vi "DAQNavi Create Channel(CO-Pulse Width).vi"(0 "task in":i32=-1, 5 "physical channels":string="DemoDevice,BID#0/cntr0", 7 "high period":dbl=-1.0, 9 "low period":dbl=-1.0, 11 "error in (no error)":errorcluster) -> (4 "task out":i32, 15 "error out":errorcluster)   [LabVIEW 2020]
uses:
  DAQNavi_LV.dll
panel:
  in  "pulse width 2":cluster{"high period":dbl, "low period":dbl}
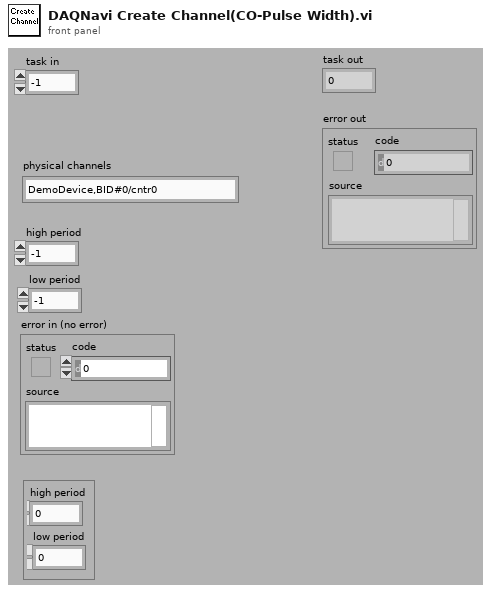
[diagram p1: front panel]
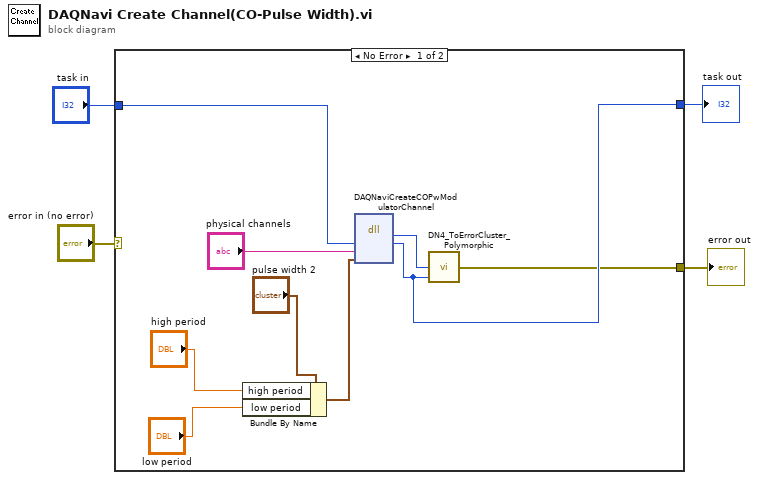
[diagram p0: block diagram]
diagram:
  n1 = case shown="No Error" "error in (no error)" {
    selector: "error in (no error)" -> [_ w14]
    tunnel: "task in" -> [w13 w15]
    tunnel: [w6 w15] -> w2
    tunnel: [w5 w14] -> w1
    frame No Error {
      n2 = Bundle By Name(cluster="pulse width 2", "high period"="high period", "low period"="low period") -> (w7:cluster{"high period":dbl, "low period":dbl})
      n3 = dll-call lib="DAQNavi_LV.dll" fn="DAQNaviCreateCOPwModulatorChannel"("taskID"=w13, "physicalChannel"="physical channels", "pulseWidth"=w7) -> ("return type"=w11:i32, "taskID"=w6:i32)  [unwired: 5 in, 2 out]
      n4 = call "DN4_ToErrorCluster_Polymorphic.vi"("task id"=w6, "error code"=w11) -> ("error out"=w5:errorcluster)  [unwired: 3 out]
    }
    frame Error {
    }
  }
  "error out" <- w1
  "task out" <- w2
